vi "indicator.vi"(8 "error_in":errorcluster, 10 "count":i32, 11 "current_num":i32) -> (0 "error_out":errorcluster, 3 "Slide":u8(slide) scale=0.0..100.0)   [LabVIEW 2017]
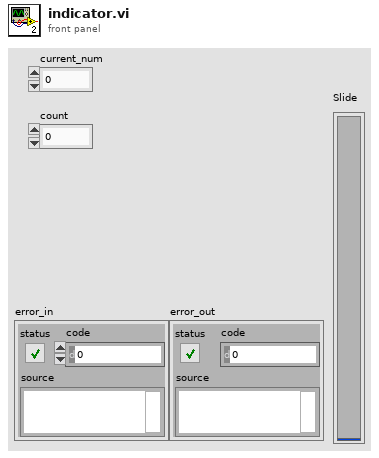
[diagram p1: front panel]
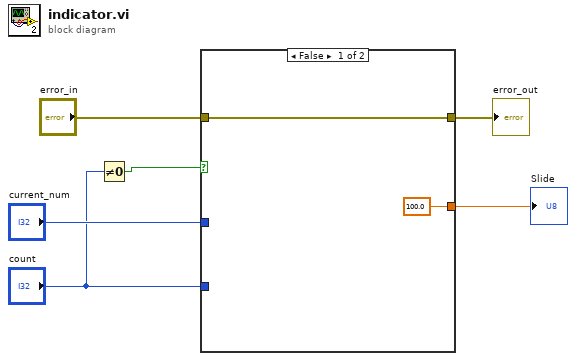
[diagram p0: block diagram]
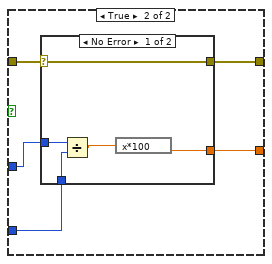
[diagram p2: hidden frame]
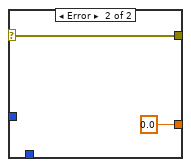
[diagram p3: hidden frame]
diagram:
  n1 = Not Equal To 0?(x="count") -> (x != 0?=w1:bool)
  n2 = case shown="False" w1 {
    tunnel: [w8 w13] -> w6
    tunnel: [100.0 w12] -> w5
    tunnel: "error_in" -> [w8 w11]
    tunnel: "current_num" -> [_ w9]
    tunnel: "count" -> [_ w10]
    frame False {
    }
    frame True {
      n3 = case shown="No Error" w11 {
        selector: w11 -> [w17 w20]
        tunnel: [w17 w20] -> w13
        tunnel: [w16 0.0] -> w12
        tunnel: w10 -> [w15 _]
        tunnel: w9 -> [w14 _]
        frame No Error {
          n4 = Divide(x=w14, y=w15) -> (x/y=w18:dbl)
          n5 = expression code="x*100"(w18) -> (w16:dbl)
        }
        frame Error {
        }
      }
    }
  }
  "error_out" <- w6
  "Slide" <- w5
